vi "实验4_2.vi"() -> ()   [LabVIEW 2018]
panel:
  in  "stop":bool
  out "Waveform Chart":cluster{"number: 0 to 1":dbl, dbl, dbl}(graph)
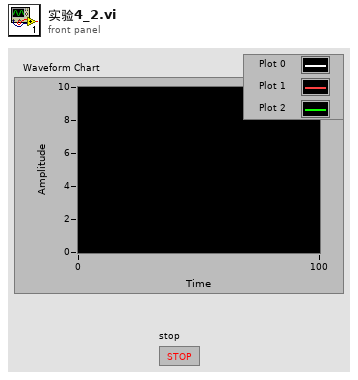
[diagram p1: front panel]
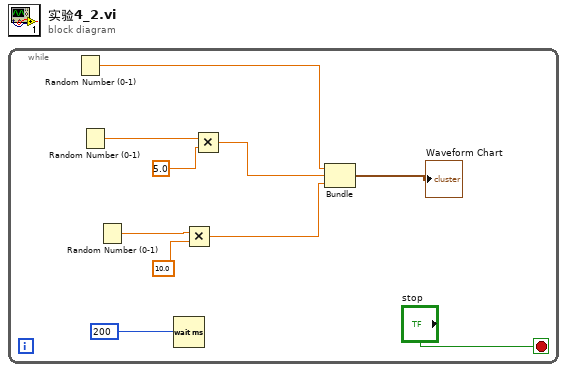
[diagram p0: block diagram]
diagram:
  n1 = while {
    stop <- "stop" stop-if-true
    n2 = Random Number (0-1)() -> (number: 0 to 1=w5:dbl)
    n3 = Random Number (0-1)() -> (number: 0 to 1=w10:dbl)
    n4 = Random Number (0-1)() -> (number: 0 to 1=w8:dbl)
    n5 = Wait (ms)(milliseconds to wait=200) -> ()  [unwired: 1 out]
    n6 = Multiply(x=w8, y=10.0) -> (x*y=w3:dbl)
    n7 = Multiply(x=w10, y=5.0) -> (x*y=w4:dbl)
    n8 = Bundle("number: 0 to 1"=w5, w4, w3) -> (→"Waveform Chart":cluster{"number: 0 to 1":dbl, dbl, dbl})  [unwired: 1 in]
  }
